vi "generator_and_acquisition.vi"() -> ()   [LabVIEW 2025]
uses:
  <vilib>/express/express analysis/Spectral/Block/exnSpectralBlock spectral measurements PSD poly.vi
  <vilib>/express/express analysis/Spectral/Block/exnSpectralBlock spectral measurements PSD WFM.vi
  <vilib>/express/express analysis/Spectral/XNode/ExpressSpectralMeasurementsBlockNode.xnode
panel:
  out "loop iteration":i32
  in  "Frequency":dbl=0.1
  out "Waveform Graph":cluster{"f0":dbl, "df":dbl, "magnitude":dbl[]}(graph)
  out "Acquisição":dynamicdata(graph)
  out "Gerador":dynamicdata(graph)
  in  "stop":bool
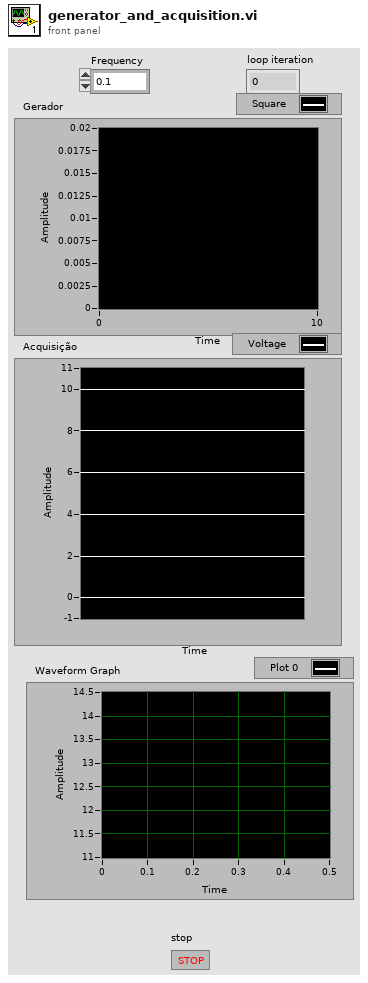
[diagram p1: front panel]
types:
  T1 = cluster{"averaging mode":u16, "weighting mode":u16, "number of averages":u32}
  T2 = cluster{"dB On (F)":bool, "unwrap phase (F)":bool, "convert to degree (F)":bool}
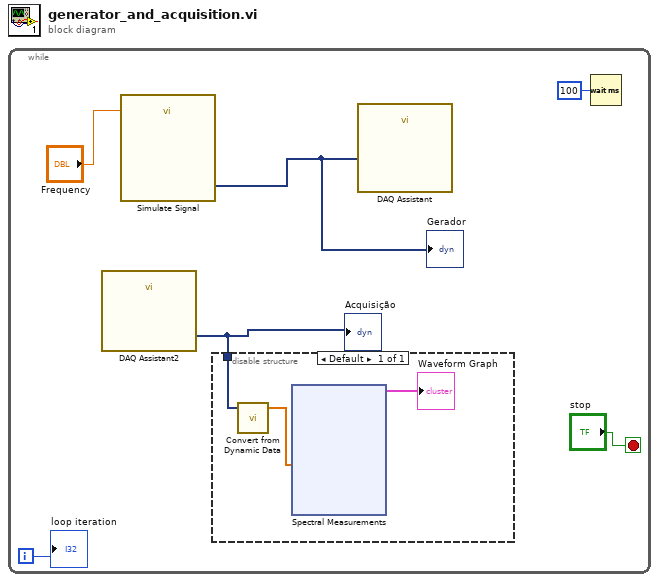
[diagram p0: block diagram]
diagram:
  n1 = while {
    i -> [w1]
    stop <- "stop" stop-if-true
    n2 = call "DAQ Assistant2"() -> ("data"=w3:dynamicdata)  [unwired: 17 in, 2 out]
    "Acquisição" <- w3
    n3 = call "Simulate Signal"("Frequency"="Frequency") -> ("Square"=w4:dynamicdata)  [unwired: 13 in, 1 out]
    "Gerador" <- w4
    n4 = disable-structure shown="Default" {
      disable-tunnel: w3 -> [w9]
      frame Enabled {
        n5 = call "Convert from Dynamic Data"("Dynamic Data Type"=w9) -> ("Array"=w8:dbl[])  [unwired: 3 in]
        n6 = xnode "Spectral Measurements"("Signals"=w8) -> ("PSD"=→"Waveform Graph":cluster{"f0":dbl, "df":dbl, "magnitude":dbl[]})  [unwired: 2 in, 2 out]
      }
    }
    n7 = call "DAQ Assistant"("data"=w4) -> ()  [unwired: 17 in, 2 out]
    n8 = Wait (ms)(milliseconds to wait=u32 100) -> ()  [unwired: 1 out]
    "loop iteration" <- w1
  }
